vi "MoveHangerPiston.vi"(11 "Arm Deploy Piston":bool) -> ()   [LabVIEW 2019]
uses:
  <vilib>/Rock Robotics/WPI/Solenoid/WPI_SolenoidValue.ctl
  <vilib>/Rock Robotics/WPI/Solenoid/Deprecated/WPI_SolenoidGetBool.vi
  <vilib>/Rock Robotics/WPI/Solenoid/WPI_SolenoidSetEnum.vi
  <vilib>/Rock Robotics/Network Tables/NT Write Boolean.vi
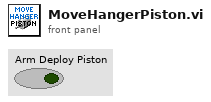
[diagram p1: front panel]
types:
  T1 = typedef "WPI_SolenoidValue.ctl" = enum16{"Off", "On", "Forward", "Reverse"}
  T2 = typedef "WPI_SolenoidDevRef.ctl" = cluster{"DevStatus":errorcluster, "Pneumatics Control Module":u8, "Forward Solenoid Channel":T3, "Reverse Solenoid Channel":T3}
  T3 = typedef "WPI_SolenoidChannel.ctl" = enum8{"Solenoid 0", "Solenoid 1", "Solenoid 2", "Solenoid 3", "Solenoid 4", "Solenoid 5", "Solenoid 6", "Solenoid 7", "Invalid"}
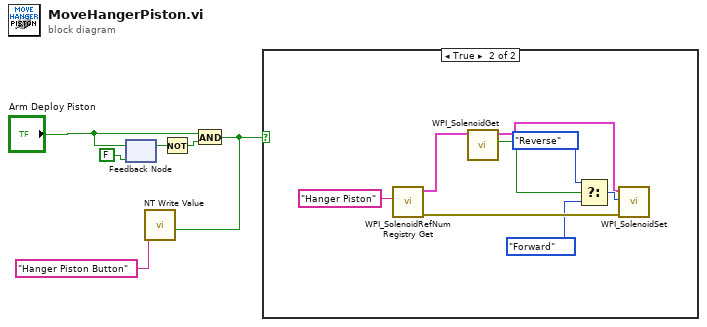
[diagram p0: block diagram]
diagram:
  n1 = feedback #1(FALSE ("Extend and Retract Arm")) -> (w5:bool)
  n2 = feedback-in #1("Arm Deploy Piston") -> ()
  n3 = Not(x=w5) -> (.not. x?=w4:bool)
  n4 = And(x="Arm Deploy Piston", y=w4) -> (x .and. y?=w1:bool)
  n5 = call-poly <vilib>:"NT Write Value.vi"("Boolean"=w1, "Name"="Hanger Piston Button") -> ()  [unwired: 9 in, 1 out]
  n6 = case shown="True" w1 {
    frame False {
    }
    frame True {
      n7 = call <vilib>:"WPI_SolenoidRefNum Registry Get.vi"("refnum name"="Hanger Piston") -> ("error out"=w13:errorcluster, "SolenoidDevRef"=w9:T2)  [unwired: 9 in]
      n8 = call-poly <vilib>:"WPI_SolenoidGet.vi"("SolenoidDevRef"=w9) -> ("Value"=w7:bool, "SolenoidDevRef"=w8:T2)  [unwired: 8 in, 1 out]
      n9 = Select(t=WPI_SolenoidValue."Reverse" ("Value"), s=w7, f=WPI_SolenoidValue."Forward" ("Value")) -> (s? t:f=w10:T1)
      n10 = call-poly <vilib>:"WPI_SolenoidSet.vi"("error in (no error)"=w13, "Value"=w10, "SolenoidDevRef"=w8) -> ()  [unwired: 7 in, 2 out]
    }
  }
